vi "MoveAngle.vi"(6 "reinitialize? (F)":bool, 9 "Angle Target":dbl) -> (1 "Done?":bool)   [LabVIEW 2013]
uses:
  <vilib>/addons/control/pid/pid.llb/PID (DBL).vi
  <vilib>/Rock Robotics/WPI/RobotDrive/WPI_RobotDriveGetSetRefNum.vi
  <vilib>/addons/control/pid/NI_PID_pid.lvlib
panel:
  in  "Adjustment Variable":dbl=0.64
  in  "PID Gains for Angle":T1={"proportional gain (Kc)"=1.2, "integral time (Ti, min)"=0.011, "derivative time (Td, min)"=0.007} {"derivative time (Td, min)" format="%.3f"; "integral time (Ti, min)" format="%.3f"; "proportional gain (Kc)" format="%.3f"}
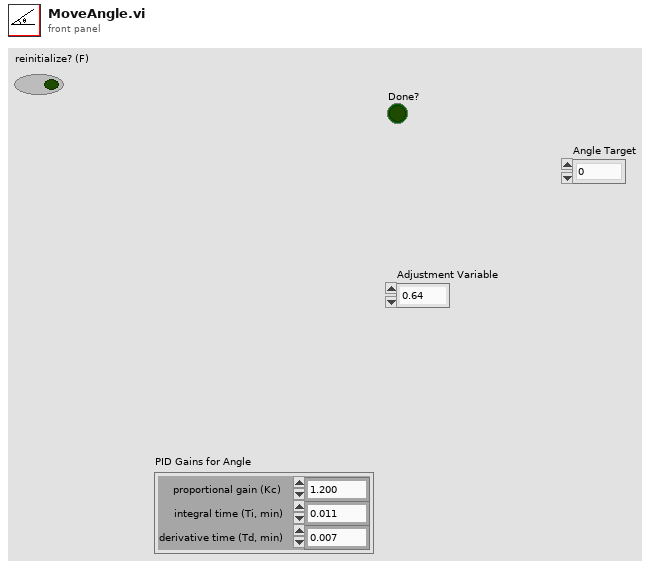
[diagram p1: front panel]
types:
  T1 = cluster{"proportional gain (Kc)":dbl, "integral time (Ti, min)":dbl, "derivative time (Td, min)":dbl}
  T2 = typedef "WPI_EncoderDevRef.ctl" = cluster{"DevStatus":errorcluster, "EncoderIndex":T3, "CounterIndex":T4, "DistancePerCount":dbl, "Decoding Type":T5}
  T3 = typedef "FPGA_EncoderIdx.ctl" = enum8{"Enc 0", "Enc 1", "Enc 2", "Enc 3", "Invalid"}
  T4 = typedef "FPGA_CounterCtrSystemIndex.ctl" = enum8{"Ctr 0", "Ctr 1", "Ctr 2", "Ctr 3", "Ctr 4", "Ctr 5", "Ctr 6", "Ctr 7", "Invalid"}
  T5 = typedef "WPI_EncoderType.ctl" = enum16{"1x", "2x", "4x"}
  T6 = typedef "WPI_RobotDriveDevRef.ctl" = cluster{"DevStatus":errorcluster, "Motors[]":T7[], "Square Inputs":bool, "Max Output":dbl, "Isochronous":bool}
  T7 = typedef "WPI_MotorControlDeviceRef.ctl" = cluster{"DeviceStatus":errorcluster, "Type":enum16{"PWM", "CAN"}, "PWM":cluster{"Digital Module":T8, "PWM Channel":T9, "DeadBand":T10}, "CAN":cluster{"Device Number":u8, "Control Mode":T11, "Semaphore":T12, "Max Vout":dbl}, "Invert":bool, "TransformRef":T13, "InvTransformRef":T13}
  T8 = typedef "FPGA_TypedefDigitalModule.ctl" = enum16{"Digital Module 1", "Digital Module 2"}
  T9 = typedef "FPGA_DIOPWMChannel.ctl" = enum8{"PWM 1", "PWM 2", "PWM 3", "PWM 4", "PWM 5", "PWM 6", "PWM 7", "PWM 8", "PWM 9", "PWM 10", "Invalid"}
  T10 = typedef "WPI_PWMDeadband.ctl" = cluster{"Name":string, "maxPositivePwm":i32, "minPositivePwm":i32, "centerPwm":i32, "maxNegativePwm":i32, "minNegativePwm":i32, "angularRange":u16}
  T11 = typedef "WPI_CANJaguar_ControlMode.ctl" = enum8{"Percent VBus", "Current", "Speed", "Position", "Voltage"}
  T12 = typedef "Semaphore RefNum" = refnum<k1>
  T13 = typedef "WPI_PWMTransform_ConPane.ctl" = refnum<vi>
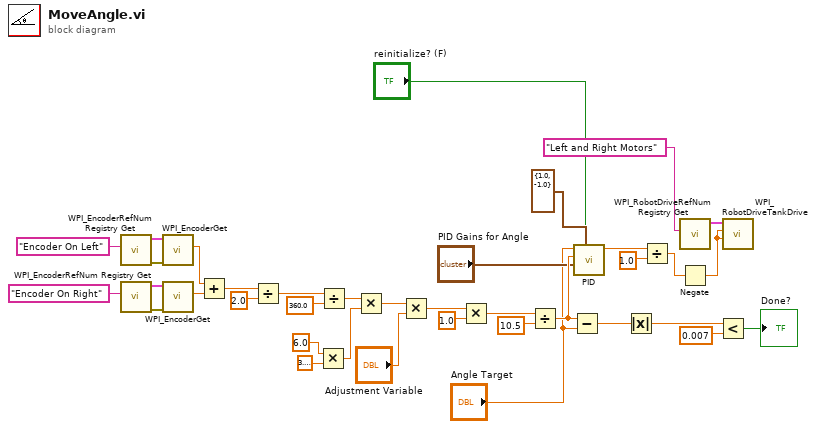
[diagram p0: block diagram]
diagram:
  n1 = call <vilib>:"WPI_EncoderRefNum Registry Get.vi"("refnum name"="Encoder On Left") -> ("error out"=w37:errorcluster, "EncoderDevRef"=w36:T2)  [unwired: 9 in]
  n2 = call <vilib>:"WPI_EncoderRefNum Registry Get.vi"("refnum name"="Encoder On Right") -> ("error out"=w35:errorcluster, "EncoderDevRef"=w34:T2)  [unwired: 9 in]
  n3 = call <vilib>:"WPI_EncoderGet.vi"("error in (no error)"=w37, "EncoderDevRef"=w36) -> ("Distance"=w31:dbl)  [unwired: 4 in, 5 out]
  n4 = call <vilib>:"WPI_EncoderGet.vi"("error in (no error)"=w35, "EncoderDevRef"=w34) -> ("Distance"=w13:dbl)  [unwired: 4 in, 5 out]
  n5 = Add(x=w31, y=w13) -> (x+y=w30:dbl)
  n6 = Divide(x=w30, y=2.0) -> (x/y=w26:dbl)
  n7 = Multiply(x=6.0, y=3.141592653589793) -> (x*y=w24:dbl)
  n8 = Divide(x=w26, y=360.0) -> (x/y=w19:dbl)
  n9 = Multiply(x=w19, y=w24) -> (x*y=w9:dbl)
  n10 = Multiply(x=w9, y="Adjustment Variable") -> (x*y=w8:dbl)
  n11 = Multiply(x=w8, y=1.0) -> (x*y=w7:dbl)
  n12 = Divide(x=w7, y=10.5) -> (x/y=w15:dbl)
  n13 = Subtract(x=w15, y="Angle Target") -> (x-y=w16:dbl)
  n14 = call-poly <vilib>:"PID.vi"("reinitialize? (F)"="reinitialize? (F)", "output range"=cluster{"output high":dbl, "output low":dbl} {"output high"=1.0, "output low"=-1.0}, "PID gains"="PID Gains for Angle", "process variable"=w15, "setpoint"="Angle Target") -> ("output"=w20:dbl)  [unwired: 5 in, 1 out]
  n15 = Absolute Value(x=w16) -> (abs(x)=w17:dbl)
  n16 = Divide(x=w20, y=1.0) -> (x/y=w12:dbl)
  n17 = call <vilib>:"WPI_RobotDriveRefNum Registry Get.vi"("refnum name"="Left and Right Motors") -> ("RobotDriveDevRef"=w21:T6)  [unwired: 9 in, 1 out]
  n18 = Negate(x=w12) -> (-x=w11:dbl)
  n19 = Less?(x=w17, y=0.007) -> (x < y?=→"Done?":bool)
  n20 = call <vilib>:"WPI_RobotDriveTankDrive.vi"("Right axis value"=w11, "Left axis value"=w11, "RobotDriveDevRef"=w21) -> ()  [unwired: 6 in, 3 out]
